vi "Config.vi"   [LabVIEW 2019]
uses:
  <vilib>/Utility/config.llb/Write Key (Double).vi
  <vilib>/Utility/config.llb/NI_LVConfig.lvlib
types:
  T1 = typedef "NI_LVConfig.lvlib/Config Data RefNum.ctl" = refnum<k1>
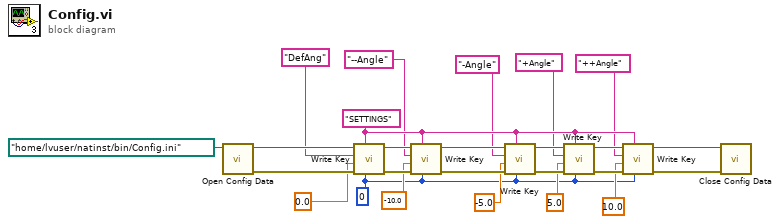
[diagram p0: block diagram]
diagram:
  w1 = i16 0 ("precision (6)")
  w12 = "SETTINGS" ("section")
  n1 = call <vilib>:"Open Config Data.vi"("configuration file path"=path "/home/lvuser/natinst/bin/Config.ini") -> ("error out"=w23:errorcluster, "refnum"=w24:T1)  [unwired: 8 in, 1 out]
  n2 = call-poly <vilib>:"Write Key.vi"("precision (6)"=w1, "section"=w12, "error in (no error)"=w23, "value"=0.0, "key"="DefAng", "refnum"=w24) -> ("error out"=w21:errorcluster, "refnum out"=w22:T1)  [unwired: 3 in, 1 out]
  n3 = call-poly <vilib>:"Write Key.vi"("precision (6)"=w1, "section"=w12, "error in (no error)"=w21, "value"=-10.0, "key"="--Angle", "refnum"=w22) -> ("error out"=w19:errorcluster, "refnum out"=w20:T1)  [unwired: 3 in, 1 out]
  n4 = call-poly <vilib>:"Write Key.vi"("precision (6)"=w1, "section"=w12, "error in (no error)"=w19, "value"=-5.0, "key"="-Angle", "refnum"=w20) -> ("error out"=w17:errorcluster, "refnum out"=w18:T1)  [unwired: 3 in, 1 out]
  n5 = call-poly <vilib>:"Write Key.vi"("precision (6)"=w1, "section"=w12, "error in (no error)"=w17, "value"=5.0, "key"="+Angle", "refnum"=w18) -> ("error out"=w15:errorcluster, "refnum out"=w16:T1)  [unwired: 3 in, 1 out]
  n6 = call-poly <vilib>:"Write Key.vi"("precision (6)"=w1, "section"=w12, "error in (no error)"=w15, "value"=10.0, "key"="++Angle", "refnum"=w16) -> ("error out"=w13:errorcluster, "refnum out"=w14:T1)  [unwired: 3 in, 1 out]
  n7 = call <vilib>:"Close Config Data.vi"("error in (no error)"=w13, "refnum"=w14) -> ()  [unwired: 8 in, 2 out]
